vi "UpdateGEKML.vi"(8 "error in":errorcluster, 10 "KML File Path In":path, 11 "GE Ref":refnum<k7>) -> (0 "error out":errorcluster, 3 "GE Ref":refnum<k7>)   [LabVIEW 2015]
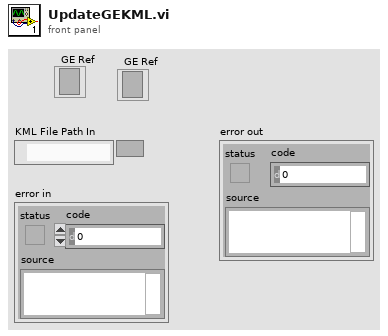
[diagram p1: front panel]
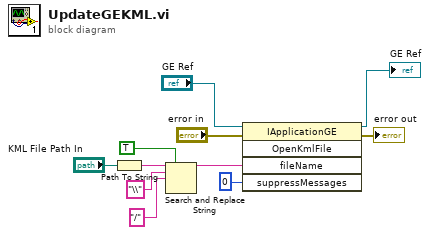
[diagram p0: block diagram]
diagram:
  n1 = Path To String(path="KML File Path In") -> (string=w6:string)
  n2 = Search and Replace String(replace all?=TRUE ("replace all? (F)"), input string=w6, search string="\\", replace string="/" ("replace string (\"\")")) -> (result string=w11:string)  [unwired: 4 in, 3 out]
  n3 = invoke class="IApplicationGE" method="OpenKmlFile"(reference="GE Ref", error in="error in", "fileName"=w11, "suppressMessages"=0) -> (reference out=→"GE Ref":refnum<k7>, error out=→"error out":errorcluster)  [unwired: 1 in, 3 out]
